vi "MT Demodulate FSK.vi"(0 "input complex waveform":T1={"t0"=0.0, "dt"=1.0, "Y"=[]} {"Y" format="%.3f"; "dt" format="%^.2e"; "t0" format="%.4f"}, 5 "FSK system parameters":T4={"samples per symbol (16)"=16, "symbol map"=[], "symbol phase continuity"=enum."continuous"} {"symbol map" format="%.2f"}, 7 "matched filter coefficients":dbl[](array[numeric]) format="%.2f", 9 "synchronization parameters":T3 {"sync sequence" format="%.2f"}, 11 "error in (no error)":errorcluster, 12 "pulse shaping filter coefficients":dbl[](array[numeric]) format="%.2f", 13 "reset? (T)":bool=TRUE) -> (4 "recovered complex waveform":T1 {"Y" format="%.3f"; "dt" format="%^.2e"; "t0" format="%.4f"}, 6 "output bit stream":i8[](array[numeric]), 8 "measurements":T2 {"FSK error (Hz)" format="%.2f"; "deviation error (Hz)" format="%.2f"; "frequency drift (Hz)" format="%.2f"; "frequency offset (Hz)" format="%.2f"}, 10 "sync found index (symbols)":dbl format="%.4f", 15 "error out":errorcluster)   [LabVIEW 2020, in "niDMT.lvlib"]
doc: "Demodulates an frequency-shift keying (FSK)-modulated complex baseband waveform and returns the time-aligned demodulated waveform, the demodulated information bit stream, and measurement results obtained during demodulation. This VI attempts to remove carrier and phase offset by locking to the carrier signal."
uses:
  <vilib>/addons/Modulation/niDMT.lvlib
  <vilib>/addons/Modulation/Analog/controls/Complex Data Waveform.ctl
  <vilib>/addons/Modulation/Analog/MT Resample (Complex Cluster).vi
  <vilib>/addons/Modulation/Analog/support/Validators/mod_Fractional Resample Validate.vi
  <vilib>/addons/Modulation/Analog/support/Validators/mod_Check Flush State.vi
  <vilib>/addons/Modulation/Analog/support/mod_FractionalResampler.vi
  <vilib>/addons/Modulation/Analog/support/mod_Integer Rate Interpolation.vi
  <vilib>/addons/Modulation/Analog/support/Validators/mod_Validate Complex Waveform.vi
  <vilib>/addons/Modulation/Analog/support/mod_PerformResampling.vi
  <vilib>/addons/Modulation/Analog/support/Validators/mod_WFErrorHandler.vi
  <vilib>/addons/Modulation/Digital/Support/Common/mod_Truncate FIR Filter (real).vi
  <vilib>/Utility/error.llb/Error Cluster From Error Code.vi
  <vilib>/addons/Modulation/Analog/support/mod_Resampling Factors.vi
  <vilib>/addons/Modulation/Analog/support/mod_ResamplingFilter.vi
  <vilib>/addons/Modulation/Analog/support/mod_Generate Integer Interpolation Filter.vi
  <vilib>/addons/Modulation/niAMT.lvlib
  <vilib>/Analysis/NI_AALBase.lvlib
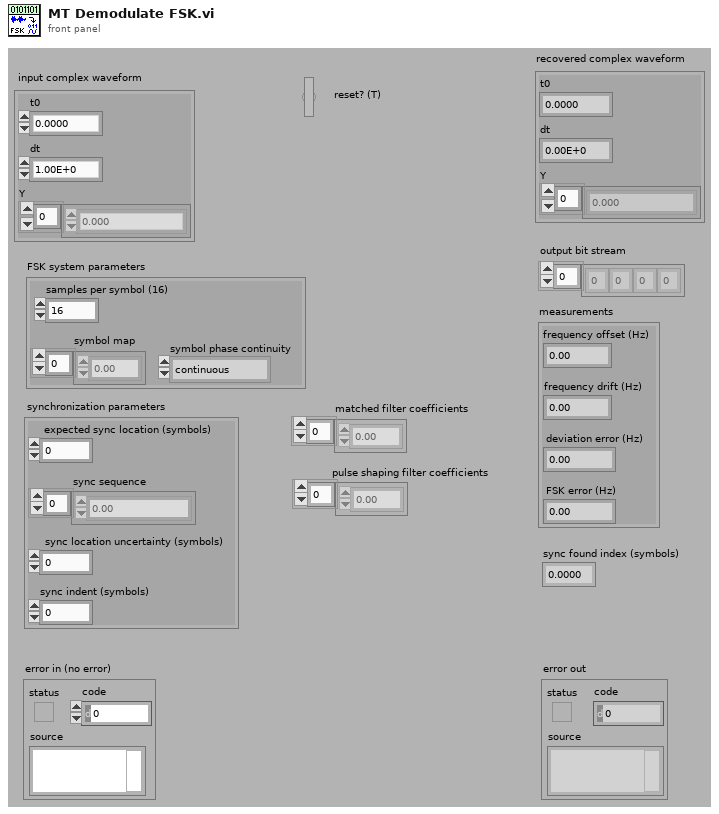
[diagram p1: front panel]
types:
  T1 = typedef "niAMT.lvlib/Complex Data Waveform.ctl" = cluster{"t0":dbl, "dt":dbl, "Y":cdb[]}
  T2 = cluster{"frequency offset (Hz)":dbl, "frequency drift (Hz)":dbl, "deviation error (Hz)":dbl, "FSK error (Hz)":dbl}
  T3 = cluster{"expected sync location (symbols)":i32, "sync sequence":cdb[], "sync location uncertainty (symbols)":i32, "sync indent (symbols)":i32}
  T4 = cluster{"samples per symbol (16)":i32, "symbol map":dbl[], "symbol phase continuity":enum16{"continuous", "discontinuous"}}
  T5 = enum16{"FSK", "PSK", "QAM", "MSK", "PAM", "ASK", "CPM"}
  T6 = cluster{dbl, "dt":dbl, "Received Signal Out":cdb[]}
  T7 = cluster{"Frequency Estimate (Hz)":dbl, "Frequency Drift (Hz)":dbl, "Deviation Error, Hz":dbl, "FSK Error, Hz":dbl}
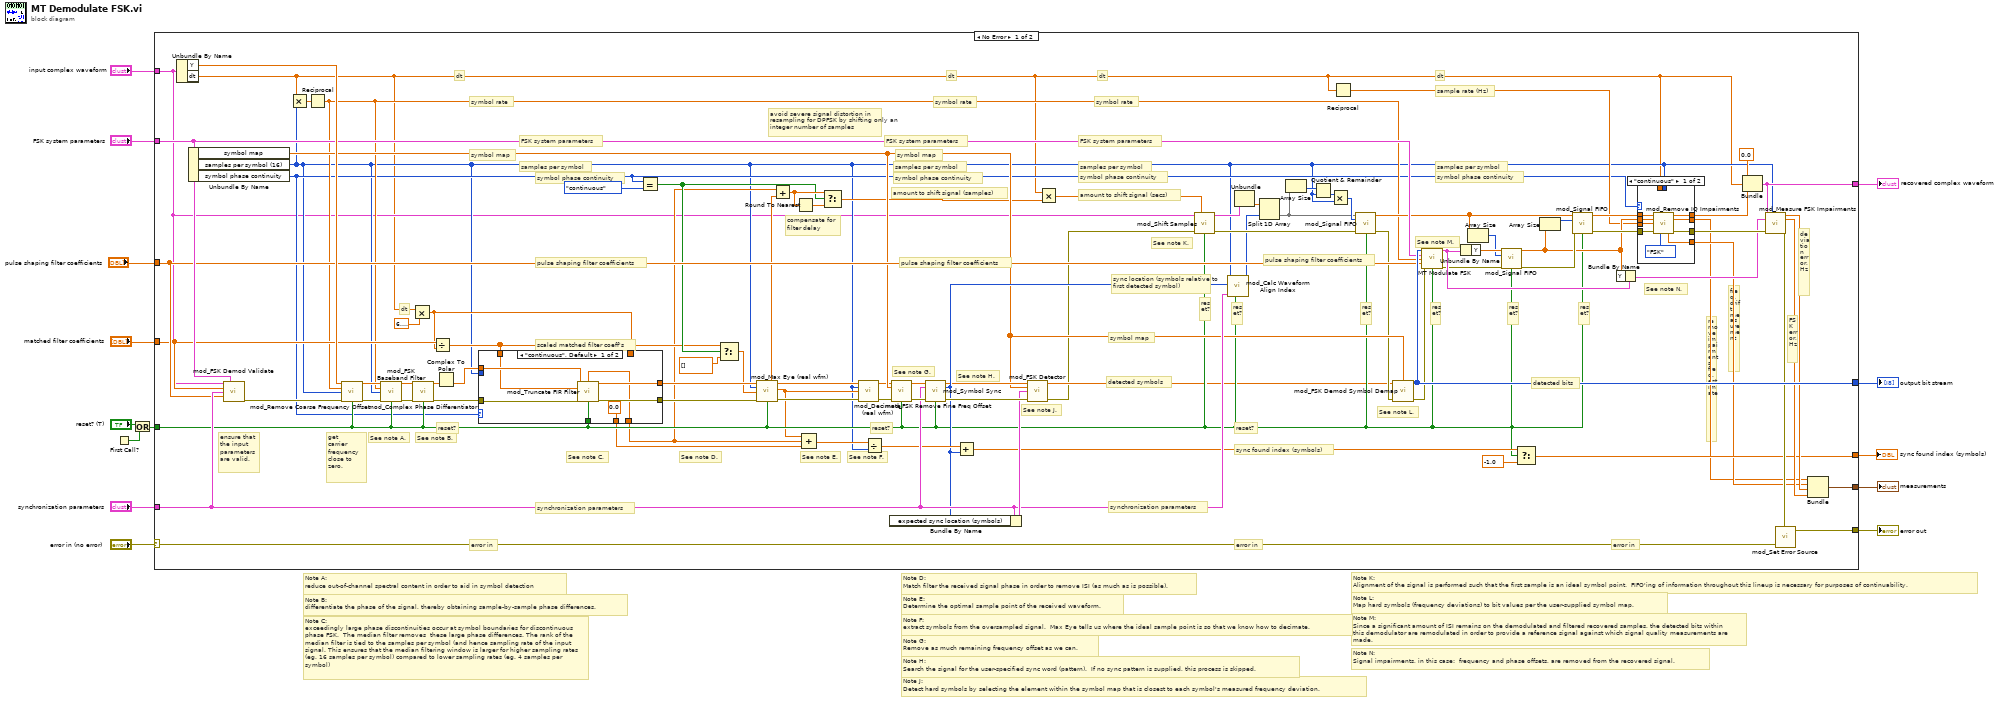
[diagram p0: block diagram]
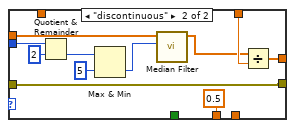
[diagram p2: hidden frame]
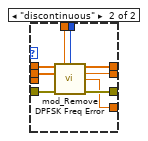
[diagram p3: hidden frame]
diagram:
  # "Note N:\nSignal impairments, in this case:  frequency and phase offsets, are removed from the recovered signal."
  # "Note M:\nSince a significant amount of ISI remains on the demodulated and filtered recovered samples, the detected bits within this demodulator are remodulated in order to provide a reference signal against which signal quality measurements are made."
  # "Note L:\nMap hard symbols (frequency deviations) to bit values per the user-supplied symbol map."
  # "Note K:\nAlignment of the signal is performed such that the first sample is an ideal symbol point.  FIFO'ing of information throughout this lineup is necessary for purposes of continuability."
  # "Note J:\nDetect hard symbols by selecting the element within the symbol map that is closest to each symbol's measured frequency deviation."
  # "Note H:\nSearch the signal for the user-specified sync word (pattern).  If no sync pattern is supplied, this process is skipped."
  # "Note G:\nRemove as much remaining frequency offset as we can."
  # "Note F:\nextract symbols from the oversampled signal.  Max Eye tells us where the ideal sample point is so that we know how to decimate."
  # "Note E:\nDetermine the optimal sample point of the received waveform."
  # "Note D:\nMatch filter the received signal phase in order to remove ISI (as much as is possible)."
  # "Note C:\nexceedingly large phase discontinuities occur at symbol boundaries for discontinuous phase FSK.  The median filter removes  these large phase differences. The rank of the \nmedian filter is tied to the samples per symbol (and hence sampling rate of the input\nsignal. This ensures that the median filtering window is larger for higher sampling rates\n(eg. 16 samples per symbol) compared to lower sampling rates (eg. 4 samples per symbol)"
  # "Note B:\ndifferentiate the phase of the signal, thereby obtaining sample-by-sample phase differences."
  # "Note A:\nreduce out-of-channel spectral content in order to aid in symbol detection"
  n1 = First Call?() -> (First Call?: T/F=w1:bool)
  n2 = Or(x="reset? (T)", y=w1) -> (x .or. y?=w2:bool)
  n3 = case shown="No Error" "error in (no error)" {
    selector: "error in (no error)" -> [w96 w142]
    tunnel: [w97 w142] -> w6
    tunnel: "synchronization parameters" -> [w82 _]
    tunnel: "matched filter coefficients" -> [w49 _]
    tunnel: "FSK system parameters" -> [w86 _]
    tunnel: "pulse shaping filter coefficients" -> [w67 _]
    tunnel: [w74 _] -> w7
    tunnel: "input complex waveform" -> [w16 _]
    tunnel: [w102 _] -> w8
    tunnel: [w100 _] -> w5
    tunnel: w2 -> [w33 _]
    tunnel: [w90 _] -> w3
    frame No Error {
      # "See note N."
      # "See note M."
      # "See note L."
      # "See note K."
      # "See note J."
      # "See note H."
      # "See note G."
      # "See note F."
      # "See note E."
      # "See note D."
      # "See note C."
      # "get\ncarrier\nfrequency \nclose to\nzero."
      # "ensure that\nthe input\nparameters\nare valid."
      # "See note B."
      # "See note A."
      # "FSK error, Hz"
      # "deviation error, Hz"
      # "avoid severe signal distortion in resampling for DPFSK by shifting only an integer number of samples"
      # "reset?"
      # "freq. drift measurement"
      # "reset?"
      # "reset?"
      # "reset?"
      # "reset?"
      # "reset?"
      # "remove impairments freq. estimate"
      # "error in"
      # "detected bits"
      # "error in"
      # "synchronization parameters"
      # "error in"
      # "synchronization parameters"
      # "sync found index (symbols)"
      # "symbol phase continuity"
      # "samples per symbol"
      # "sample rate (Hz)"
      # "dt"
      # "reset?"
      # "reset?"
      # "reset?"
      # "detected symbols"
      # "sync location (symbols relative to first detected symbol)"
      # "pulse shaping filter coefficients"
      # "amount to shift signal (secs)"
      # "symbol map"
      # "symbol rate"
      # "dt"
      # "FSK system parameters"
      # "symbol map"
      # "samples per symbol"
      # "symbol phase continuity"
      # "symbol rate"
      # "dt"
      # "FSK system parameters"
      # "samples per symbol"
      # "symbol phase continuity"
      # "pulse shaping filter coefficients"
      # "amount to shift signal (samples)"
      # "scaled matched filter coeff's"
      # "pulse shaping filter coefficients"
      # "symbol phase continuity"
      # "samples per symbol"
      # "compensate for filter delay"
      # "symbol map"
      # "FSK system parameters"
      # "dt"
      # "dt"
      # "symbol rate"
      n4 = Unbundle By Name(w16) -> ("Y"=w99:cdb[], "dt"=w15:dbl)
      n5 = Unbundle By Name(w86) -> ("symbol map"=w52:dbl[], "samples per symbol (16)"=w18:i32, "symbol phase continuity"=w20:enum16{"continuous", "discontinuous"})
      n6 = call <vilib>:"mod_FSK Demod Validate.vi"("Input Complex Waveform"=w16, "FSK System Parameters"=w86, "Matched Filter Coefficients"=w49, "Synchronization Parameters"=w82, "Pulse Shaping Filter Coefficients"=w67) -> ("error out"=w87:errorcluster)  [unwired: 10 out]
      n7 = Multiply(x=w15, y=w18) -> (x*y=w101:dbl)
      n8 = Reciprocal(x=w101) -> (1/x=w32:dbl)
      n9 = call <vilib>:"mod_Remove Coarse Frequency Offset.vi"("Signal In"=w99, "Symbol Rate, Hz"=w32, "Samples Per Symbol (16)"=w18, "error in (no error)"=w87, "Reset? (T)"=w33) -> ("Signal Out"=w34:cdb[], "error out"=w35:errorcluster)  [unwired: 9 out]
      n10 = call <vilib>:"mod_FSK Baseband Filter.vi"("Signal In"=w34, "Symbol Rate, Hz"=w32, "Samples Per Symbol (16)"=w18, "error in (no error)"=w35, "Reset? (T)"=w33) -> ("Signal Out"=w37:cdb[], "error out"=w36:errorcluster)  [unwired: 9 in]
      n11 = Multiply(x=w15, y=6.283185307179586) -> (x*y=w30:dbl)
      n12 = call <vilib>:"mod_Complex Phase Differentiator.vi"("Signal In"=w37, "error in (no error)"=w36, "Reset? (T)"=w33) -> ("Signal Out"=w56:cdb[], "error out"=w21:errorcluster)  [unwired: 11 out]
      n13 = Divide(x=w49, y=w30) -> (x/y=w28:dbl[])
      n14 = Complex To Polar(r * e^(i*theta)=w56) -> (theta=w22:dbl[])  [unwired: 1 out]
      n15 = case shown="\"continuous\", Default" w20 {
        tunnel: [w112 w121] -> w54
        tunnel: [w111 w122] -> w53
        tunnel: [w110 _] -> w24
        tunnel: w22 -> [w109 w116]
        tunnel: w28 -> [w108 _]
        tunnel: w21 -> [w107 w121]
        tunnel: w33 -> [w106 _]
        tunnel: w30 -> [_ w123]
        tunnel: w18 -> [_ w114]
        tunnel: [0.0 0.5] -> w19
        frame "continuous", Default {
          n16 = call-poly <vilib>:"mod_Truncate FIR Filter.vi"("Signal In"=w109, "Filter Coefficients"=w108, "error in (no error)"=w107, "Reset? (T)"=w106) -> ("Fractional Delay (samples)"=w110:dbl, "Signal Out"=w111:dbl[], "error out"=w112:errorcluster)  [unwired: 8 in, 1 out]
        }
        frame "discontinuous" {
          n17 = Quotient & Remainder(x=w114, y=2) -> (floor(x/y)=w119:i32)  [unwired: 1 out]
          n18 = Max & Min(x=w119, y=5) -> (min(x,y)=w117:i32)  [unwired: 1 out]
          n19 = call <vilib>:"Median Filter.vi"("left rank"=w117, "X"=w116) -> ("Filtered X"=w115:dbl[])  [unwired: 1 in, 8 out]
          n20 = Divide(x=w115, y=w123) -> (x/y=w122:dbl[])
        }
      }
      n21 = Equal?(x=w20, y=enum16{"continuous", "discontinuous"}."continuous") -> (x = y?=w29:bool)
      n22 = Select(t=w28, s=w29, f=dbl[] []) -> (s? t:f=w26:dbl[])
      n23 = call <vilib>:"mod_Max Eye (real wfm).vi"("Signal In"=w53, "Samples Per Symbol (16)"=w18, "Filter Coefficients"=w26, "error in (no error)"=w54, "Reset? (T)"=w33) -> ("Waveform Alignment Offset"=w51:dbl, "Signal Out"=w57:dbl[], "Optimal Offset (samples)"=w25:dbl, "error out"=w103:errorcluster)  [unwired: 6 in, 1 out]
      n24 = Add(x=w24, y=w51) -> (x+y=w42:dbl)
      n25 = Round To Nearest(number=w42) -> (nearest integer value=w41:dbl)
      n26 = Compound Arithmetic op=ADD(w25, w24, w19) -> (w23:dbl)
      n27 = Select(t=w42, s=w29, f=w41) -> (s? t:f=w44:dbl)
      n28 = call <vilib>:"mod_Decimate (real wfm).vi"("Signal In"=w57, "Samples Per Symbol (16)"=w18, "Offset"=w25, "error in (no error)"=w103) -> ("Signal Out"=w50:dbl[], "error out"=w85:errorcluster)  [unwired: 10 in]
      n29 = Divide(x=w23, y=w18) -> (x/y=w77:dbl)
      n30 = call <vilib>:"mod_FSK Remove Fine Freq Offset.vi"("Symbols"=w50, "Symbol Map"=w52, "error in (no error)"=w85, "Reset? (T)"=w33) -> ("Symbols"=w83:dbl[], "error out"=w84:errorcluster)  [unwired: 1 in, 9 out]
      n31 = call <vilib>:"mod_Symbol Sync.vi"("Signal In"=w83, "Synchronization Parameters"=w82, "error in (no error)"=w84, "Reset? (T)"=w33) -> ("Signal Out"=w55:cdb[], "Sync Location (symbols)"=w76:i32, "error out"=w104:errorcluster)  [unwired: 9 out]
      n32 = Bundle By Name(cluster=w82, "expected sync location (symbols)"=w76) -> (w98:T3)
      n33 = Add(x=w77, y=w76) -> (x+y=w73:dbl)
      n34 = call <vilib>:"mod_FSK Detector.vi"("Symbols"=w55, "Symbol Map"=w52, "Synchronization Parameters"=w98, "error in (no error)"=w104) -> ("Detected Symbols"=w31:dbl[], "error out"=w17:errorcluster)  [unwired: 1 in, 9 out]
      n35 = Multiply(x=w15, y=w44) -> (x*y=w60:dbl)
      n36 = call <vilib>:"mod_Shift Samples.vi"("Input Complex Waveform"=w16, "Initial Sample Offset, sec"=w60, "error in (no error)"=w17, "Reset? (T)"=w33) -> ("Output Complex Waveform"=w46:T1, "error out"=w68:errorcluster)  [unwired: 10 in]
      n37 = call <vilib>:"mod_Calc Waveform Align Index.vi"("Reset? (T)"=w33, "Synchronization Parameters"=w82, "Sync Location, symbols"=w76, "Samples Per Symbol (16)"=w18) -> ("align index, samples"=w59:i32)  [unwired: 7 out]
      n38 = Unbundle(w46) -> ("Y"=w58:cdb[])  [unwired: 2 out]
      n39 = Split 1D Array(array=w58, index=w59) -> (second subarray=w69:cdb[])  [unwired: 1 out]
      n40 = Array Size(array=w69) -> (size(s)=w72:i32)
      n41 = Quotient & Remainder(x=w72, y=w18) -> (floor(x/y)=w71:i32)  [unwired: 1 out]
      n42 = Multiply(x=w71, y=w18) -> (x*y=w70:i32)
      n43 = Reciprocal(x=w15) -> (1/x=w47:dbl)
      n44 = call <vilib>:"mod_Signal FIFO.vi"("Signal In"=w69, "Output Length"=w70, "error in (no error)"=w68, "Reset? (T)"=w33) -> ("Signal Out"=w40:cdb[], "error out"=w38:errorcluster)  [unwired: 10 out]
      n45 = call <vilib>:"mod_FSK Demod Symbol Demap.vi"("Symbols In"=w31, "Symbol Map"=w52, "error in (no error)"=w38) -> ("Bits Out"=w102:i8[], "error out"=w81:errorcluster)  [unwired: 11 out]
      n46 = call <vilib>:"MT Modulate FSK.vi"("input bit stream"=w102, "FSK system parameters"=w86, "symbol rate (Hz)"=w32, "pulse shaping filter coefficients"=w67, "error in (no error)"=w81, "reset? (T)"=w33) -> ("output complex waveform"=w92:T1, "error out"=w79:errorcluster)  [unwired: 1 in, 7 out]
      n47 = Unbundle By Name(w92) -> ("Y"=w80:cdb[])
      n48 = Array Size(array=w40) -> (size(s)=w78:i32)
      n49 = call <vilib>:"mod_Signal FIFO.vi"("Signal In"=w80, "Output Length"=w78, "error in (no error)"=w79, "Reset? (T)"=w33) -> ("Signal Out"=w61:cdb[], "error out"=w64:errorcluster)  [unwired: 10 out]
      n50 = Select(t=w73, s=w33, f=-1.0) -> (s? t:f=w74:dbl)
      n51 = Array Size(array=w61) -> (size(s)=w65:i32)
      n52 = call <vilib>:"mod_Signal FIFO.vi"("Signal In"=w40, "Output Length"=w65, "error in (no error)"=w64, "Reset? (T)"=w33) -> ("Signal Out"=w62:cdb[], "error out"=w63:errorcluster)  [unwired: 10 out]
      n53 = Bundle By Name(cluster=w92, "Y"=w61) -> (w91:T1)
      n54 = case shown="\"continuous\"" w20 {
        tunnel: w47 -> [w132 _]
        tunnel: [w131 w134] -> w39
        tunnel: w62 -> [w130 w135]
        tunnel: [w129 w139] -> w95
        tunnel: [w128 w136] -> w93
        tunnel: w61 -> [w127 w141]
        tunnel: w63 -> [w126 w140]
        tunnel: [w125 w133] -> w66
        tunnel: w18 -> [_ w138]
        tunnel: w15 -> [_ w137]
        frame "continuous" {
          n55 = call <vilib>:"mod_Remove IQ Impairments.vi"("Received Signal In"=w130, "Reference Signal"=w127, "Signal Rate, Hz"=w132, "error in (no error)"=w126, "Modulation Type"=T5."FSK") -> ("Received Signal Out"=w128:cdb[], "Frequency Estimate, Hz"=w131:dbl, "Frequency Drift, Hz"=w125:dbl, "error out"=w129:errorcluster)  [unwired: 1 in, 6 out]
        }
        frame "discontinuous" {
          n56 = call <vilib>:"mod_Remove DPFSK Freq Error.vi"("Received Signal In"=w135, "dt (sec)"=w137, "samples per symbol (16)"=w138, "Reference Signal"=w141, "error in (no error)"=w140) -> ("Received Signal Out"=w136:cdb[], "Frequency Estimate (Hz)"=w134:dbl, "Frequency Drift (Hz)"=w133:dbl, "error out"=w139:errorcluster)  [unwired: 7 out]
        }
      }
      n57 = Bundle(0.0, "dt"=w15, "Received Signal Out"=w93) -> (w90:T6)  [unwired: 1 out]
      n58 = call <vilib>:"mod_Measure FSK Impairments.vi"("Recovered Complex Waveform"=w90, "Samples Per Symbol (16)"=w18, "Detected Complex Waveform"=w91, "error in (no error)"=w95) -> ("Deviation Error, Hz"=w89:dbl, "FSK Error, Hz"=w88:dbl, "error out"=w94:errorcluster)  [unwired: 1 in, 8 out]
      n59 = call <vilib>:"mod_Set Error Source.vi"("initial error in (no error)"=w96, "final error in (no error)"=w94) -> ("error out"=w97:errorcluster)  [unwired: 3 out]
      n60 = Bundle("Frequency Estimate (Hz)"=w39, "Frequency Drift (Hz)"=w66, "Deviation Error, Hz"=w89, "FSK Error, Hz"=w88) -> (w100:T7)  [unwired: 1 out]
    }
    frame Error {
    }
  }
  "error out" <- w6
  "sync found index (symbols)" <- w7
  "output bit stream" <- w8
  "measurements" <- w5
  "recovered complex waveform" <- w3
